vi "Create Read Event.vi"(8 "error in":errorcluster, 11 "Win32 Event in":refnum<class "Win32 Event.lvclass">) -> (0 "error out":errorcluster, 3 "Win32 Event out":refnum<class "Win32 Event.lvclass">)   [LabVIEW 2018, in "PCANBasic.lvlib" / "Win32 Event.lvclass"]
doc: "If the function succeeds, the return value is a handle to the event object."
uses:
  Win32 Event.lvclass
  Win32 Event.lvclass/Win32 Event.ctl
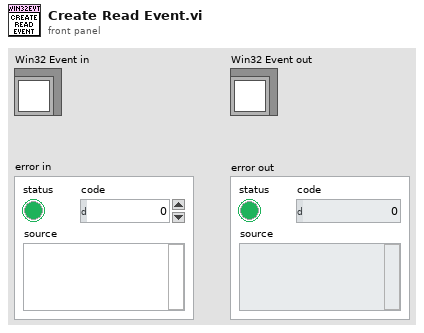
[diagram p1: front panel]
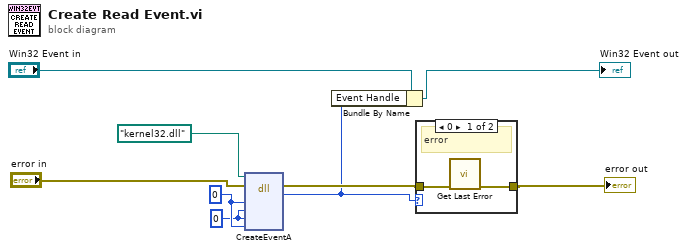
[diagram p0: block diagram]
diagram:
  w3 = 0 ("lpName")
  w4 = u64 0 ("lpName")
  n1 = dll-call lib="?" fn="CreateEventA"(path in=path "kernel32.dll", error in="error in", "lpEventAttributes"=w4, "bManualReset"=w3, "bInitialState"=w3, "lpName"=w4) -> (error out=w2:errorcluster, "hdlEvent"=w1:u64)  [unwired: 5 in, 1 out]
  n2 = Bundle By Name(cluster="Win32 Event in", "Event Handle"=w1) -> (→"Win32 Event out":refnum<class "Win32 Event.lvclass">)
  n3 = case "success?" shown="0" w1 {
    tunnel: w2 -> [w11 w12]
    tunnel: [w10 w12] -> w8
    frame 0 {
      # "error"
      n4 = call "Get Last Error.vi"("error in"=w11) -> ("error out"=w10:errorcluster)  [unwired: 10 in]
    }
    frame Default {
      # "successfull"
    }
  }
  "error out" <- w8
